vi "Create-Traj-Benchmark.vi"() -> ()   [LabVIEW 2019]
uses:
  <vilib>/Rock Robotics/WPI/ThirdParty/JAS_Junk/TrajLib/TRAJECTORY_SPLINE_TYPE_ENUM.ctl
  <vilib>/Rock Robotics/WPI/ThirdParty/JAS_Junk/TrajLib/Translation_Create.vi
  <vilib>/Rock Robotics/WPI/ThirdParty/JAS_Junk/TrajLib/Rotation_CreateAngle.vi
  <vilib>/Rock Robotics/WPI/ThirdParty/JAS_Junk/TrajLib/Trajectory_Library.lvlib
panel:
  out "Quintic Time MS":dbl format="%18.3f"
  out "Cubic Time MS":dbl format="%18.3f"
  out "XY Graph":cluster{dbl[], dbl[]}[](graph)
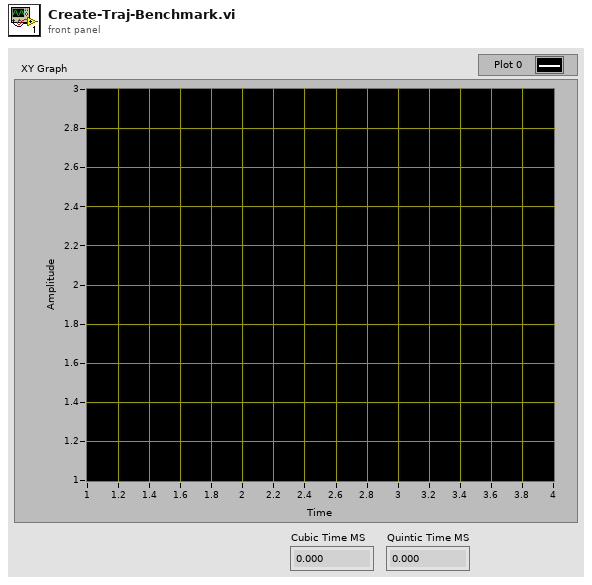
[diagram p1: front panel]
types:
  T1 = typedef "Trajectory_Library.lvlib/TRAJ_CONFIG.ctl" = cluster{"MaxVelocity":dbl, "Max Acceleration":dbl, "StartVelocity":dbl, "End Velocity":dbl, "Reversed":bool, "DiffDrKineConstntDefined":bool, "CentAcellConstntDefined":bool, "DiffDrVoltConstntDefined":bool, "DIFF_DRIVE_KINE_CONSTRAINT":T2, "CENTRIPETAL_ACCEL_CONSTRAINT":T4, "SwerveDrKineConstntDefined":bool, "SWERVE_DRIVE_KINE_CONSTRAINT":T5, "DIFF_DRIVE_VOLTAGE_CONSTRAINT":T9, "MECANUM_DRIVE_KINE_CONSTRAINT":T11, "MecanumDrKineConstntDefined":bool}
  T2 = typedef "Trajectory_Library.lvlib/TRAJ_CONSTRAINT_DIIF_DRIVE_KINEMATICS.ctl" = cluster{"Max Speed (M/S)":dbl, "DIFF_DRIVE_KINEMATICS":T3, "Max Accel (M/S2)":dbl}
  T3 = typedef "Trajectory_Library.lvlib/DIFF_DRIVE_KINEMATICS.ctl" = cluster{"TrackWidth_Meters":dbl}
  T4 = typedef "Trajectory_Library.lvlib/TRAJ_CONSTRAINT_CENTRIPETAL_ACCEL.ctl" = cluster{"Max Cent Accel":dbl}
  T5 = typedef "Trajectory_Library.lvlib/TRAJ_CONSTRAINT_SWERVE_DRIVE_KINEMATICS.ctl" = cluster{"Max Speed (M/S)":dbl, "SwerveKinematics":T6}
  T6 = typedef "Trajectory_Library.lvlib/SWERVE_DRIVE_KINEMATICS.ctl" = cluster{"NumModules":i32, "InverseKinematics":T7, "ForwardKinematics":T7, "Modules":T8[], "PrevCoR":T8}
  T7 = typedef "NI_Matrix.lvlib/RealMatrix.ctl" = dbl[][]
  T8 = typedef "Trajectory_Library.lvlib/TRANSLATION2D.ctl" = cluster{"X":dbl, "Y":dbl}
  T9 = typedef "Trajectory_Library.lvlib/TRAJ_CONSTRAINT_DIIF_DRIVE_VOLTAGE.ctl" = cluster{"Max Voltage":dbl, "DIFF_DRIVE_KINEMATICS":T3, "SIMPLE_MOTOR_FF":T10}
  T10 = typedef "Trajectory_Library.lvlib/SIMPLE_MOTOR_FF.ctl" = cluster{"Ks":dbl, "Kv":dbl, "Ka":dbl}
  T11 = typedef "Trajectory_Library.lvlib/TRAJ_CONSTRAINT_MECA_DRIVE_KINEMATICS.ctl" = cluster{"Max Speed (M/S)":dbl, "MECA_DRIVE_KINEMATICS":T12}
  T12 = typedef "Trajectory_Library.lvlib/MECA_DRIVE_KINEMATICS.ctl" = cluster{"FrontLeft":T8, "FrontRight":T8, "RearLeft":T8, "RearRight":T8, "InverseKinematics":T7, "ForwardKinematics":T7, "PrevCoR":T8}
  T13 = typedef "Trajectory_Library.lvlib/TRAJECTORY_SPLINE_TYPE_ENUM.ctl" = enum16{"Cubic", "Cubic With Weights", "Quintic", "Quintic With Weights"}
  T14 = typedef "Trajectory_Library.lvlib/WEIGHTED_WAYPOINT.ctl" = cluster{"TRANSLATION":T8, "ROTATION":T15, "SCALAR":dbl}
  T15 = typedef "Trajectory_Library.lvlib/ROTATION2D.ctl" = cluster{"VALUE":dbl, "COS":dbl, "SIN":dbl}
  T16 = typedef "Trajectory_Library.lvlib/TRAJECTORY.ctl" = cluster{"TotalTImeSecs":dbl, "States":T17[]}
  T17 = typedef "Trajectory_Library.lvlib/TRAJ_STATE.ctl" = cluster{"TimeSeconds":dbl, "Velocity":dbl, "Acceleration":dbl, "POSE":T18, "Curvature":dbl}
  T18 = typedef "Trajectory_Library.lvlib/POSE2D.ctl" = cluster{"TRANSLATION":T8, "ROTATION":T15}
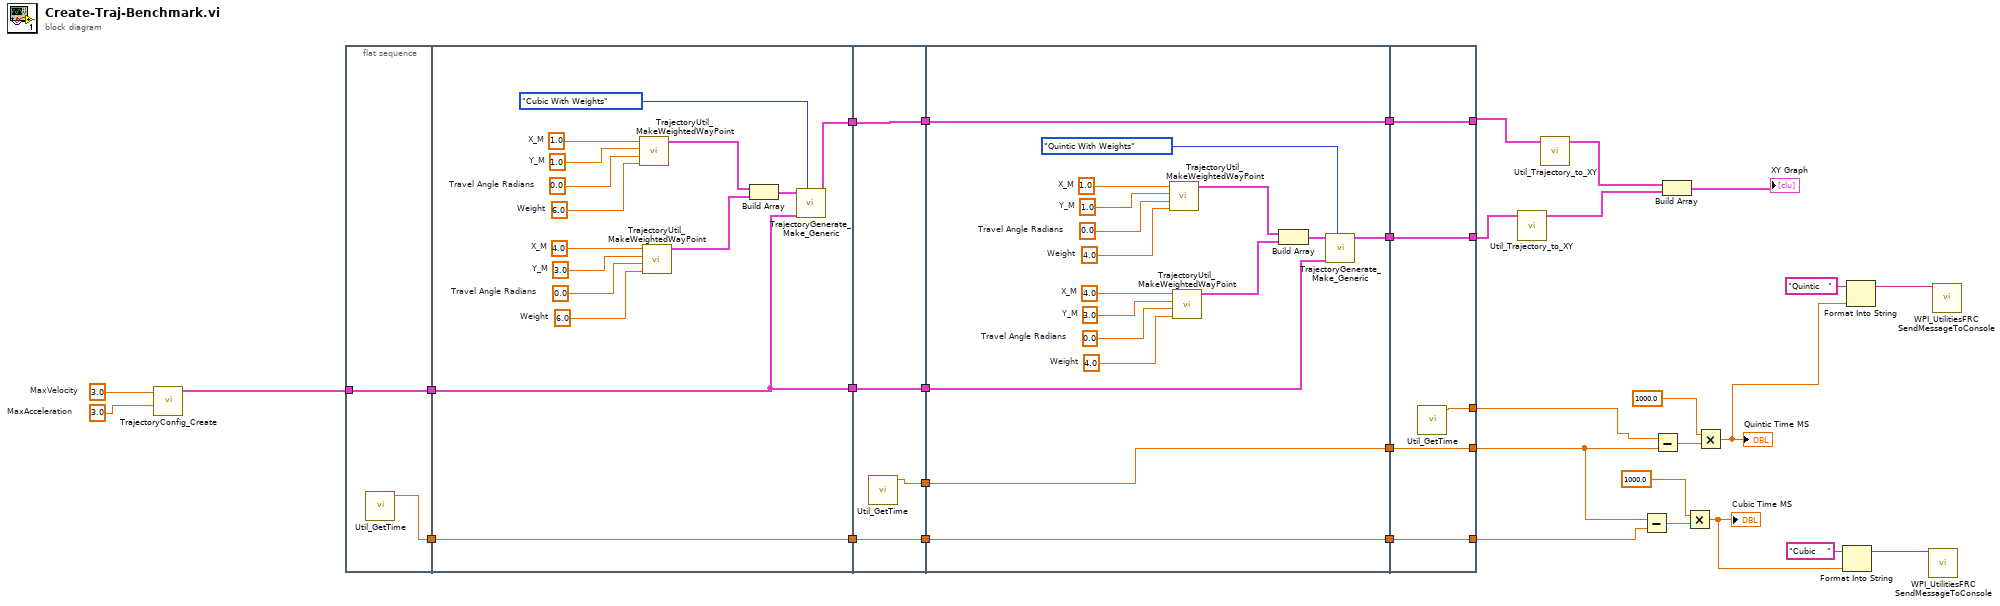
[diagram p0: block diagram]
diagram:
  w27 = 3.0  # MaxVelocity
  w28 = 3.0  # MaxAcceleration
  n1 = call <vilib>:"TrajectoryConfig_Create.vi"("MaxAcceleration"=w28, "MaxVelocity"=w27) -> ("TRAJECTORY_CONFIG"=w25:T1)  [unwired: 9 in]
  n2 = flat-sequence {
    tunnel: [w36] -> w32
    tunnel: [w35] -> w26
    tunnel: w25 -> [w35]
    tunnel: [w40] -> w33
    tunnel: w32 -> [w39]
    tunnel: [w39] -> w31
    tunnel: w26 -> [w37]
    tunnel: [w37] -> w21
    tunnel: w33 -> [w55]
    tunnel: w31 -> [w52]
    tunnel: [w55] -> w24
    tunnel: [w54] -> w23
    tunnel: [w53] -> w22
    tunnel: w21 -> [w53]
    tunnel: [w52] -> w12
    tunnel: w24 -> [w72]
    tunnel: w23 -> [w58]
    tunnel: w22 -> [w59]
    tunnel: [w72] -> w20
    tunnel: [w58] -> w16
    tunnel: [w57] -> w13
    tunnel: w12 -> [w57]
    tunnel: [w56] -> w10
    tunnel: [w77] -> w34
    tunnel: w20 -> [w77]
    tunnel: [w76] -> w17
    tunnel: [w75] -> w15
    tunnel: w16 -> [w75]
    tunnel: [w74] -> w14
    tunnel: w13 -> [w74]
    tunnel: [w73] -> w11
    tunnel: w10 -> [w73]
    frame #0 {
      n3 = call <vilib>:"Util_GetTime.vi"() -> ("FPGA_Time_Seconds"=w36:dbl)  [unwired: 10 in, 1 out]
    }
    frame #1 {
      w51 = 4.0  # X_M
      w50 = 3.0  # Y_M
      w49 = 0.0  # Travel Angle Radians
      w48 = 6.0  # Weight
      w47 = 1.0  # X_M
      w46 = 1.0  # Y_M
      w45 = 0.0  # Travel Angle Radians
      w44 = 6.0  # Weight
      n4 = call <vilib>:"TrajectoryUtil_MakeWeightedWayPoint.vi"("Weight"=w44, "Travel Angle Radians"=w45, "Y_M"=w46, "X_M"=w47) -> ("WEIGHTED_WAYPOINT"=w42:T14)  [unwired: 7 in]
      n5 = call <vilib>:"TrajectoryUtil_MakeWeightedWayPoint.vi"("Weight"=w48, "Travel Angle Radians"=w49, "Y_M"=w50, "X_M"=w51) -> ("WEIGHTED_WAYPOINT"=w41:T14)  [unwired: 7 in]
      n6 = Build Array(w42, w41) -> (w43:T14[])
      n7 = call <vilib>:"TrajectoryGenerate_Make_Generic.vi"("Spline Type"=TRAJECTORY_SPLINE_TYPE_ENUM."Cubic With Weights", "traj_config"=w37, "WeightedWayPoints"=w43) -> ("TRAJECTORY"=w40:T16)  [unwired: 7 in, 1 out]
    }
    frame #2 {
      n8 = call <vilib>:"Util_GetTime.vi"() -> ("FPGA_Time_Seconds"=w54:dbl)  [unwired: 10 in, 1 out]
    }
    frame #3 {
      w71 = 4.0  # X_M
      w70 = 3.0  # Y_M
      w69 = 0.0  # Travel Angle Radians
      w68 = 4.0  # Weight
      w67 = 1.0  # X_M
      w66 = 1.0  # Y_M
      w65 = 0.0  # Travel Angle Radians
      w64 = 4.0  # Weight
      n9 = call <vilib>:"TrajectoryUtil_MakeWeightedWayPoint.vi"("Weight"=w64, "Travel Angle Radians"=w65, "Y_M"=w66, "X_M"=w67) -> ("WEIGHTED_WAYPOINT"=w62:T14)  [unwired: 7 in]
      n10 = call <vilib>:"TrajectoryUtil_MakeWeightedWayPoint.vi"("Weight"=w68, "Travel Angle Radians"=w69, "Y_M"=w70, "X_M"=w71) -> ("WEIGHTED_WAYPOINT"=w61:T14)  [unwired: 7 in]
      n11 = Build Array(w62, w61) -> (w63:T14[])
      n12 = call <vilib>:"TrajectoryGenerate_Make_Generic.vi"("Spline Type"=TRAJECTORY_SPLINE_TYPE_ENUM."Quintic With Weights", "traj_config"=w59, "WeightedWayPoints"=w63) -> ("TRAJECTORY"=w56:T16)  [unwired: 7 in, 1 out]
    }
    frame #4 {
      n13 = call <vilib>:"Util_GetTime.vi"() -> ("FPGA_Time_Seconds"=w76:dbl)  [unwired: 10 in, 1 out]
    }
  }
  n14 = call <vilib>:"Util_Trajectory_to_XY.vi"("TRAJECTORY"=w11) -> ("outArrayXY"=w8:cluster{dbl[], dbl[]})  [unwired: 10 in]
  n15 = call <vilib>:"Util_Trajectory_to_XY.vi"("TRAJECTORY"=w34) -> ("outArrayXY"=w9:cluster{dbl[], dbl[]})  [unwired: 10 in]
  n16 = Subtract(x=w15, y=w14) -> (x-y=w30:dbl)
  n17 = Subtract(x=w17, y=w15) -> (x-y=w19:dbl)
  n18 = Build Array(w9, w8) -> (→"XY Graph":cluster{dbl[], dbl[]}[])
  n19 = Multiply(x=1000.0, y=w30) -> (x*y=w1:dbl)
  "Cubic Time MS" <- w1
  n20 = Multiply(x=1000.0, y=w19) -> (x*y=w5:dbl)
  "Quintic Time MS" <- w5
  n21 = Format Into String(initial string="Cubic    ", w1) -> (resulting string=w2:string)  [unwired: 2 in, 1 out]
  n22 = Format Into String(initial string="Quintic   ", w5) -> (resulting string=w4:string)  [unwired: 2 in, 1 out]
  n23 = call <vilib>:"WPI_UtilitiesFRC SendMessageToConsole.vi"("Message"=w2) -> ()  [unwired: 14 in, 1 out]
  n24 = call <vilib>:"WPI_UtilitiesFRC SendMessageToConsole.vi"("Message"=w4) -> ()  [unwired: 14 in, 1 out]
